vi "Tiempo.vi"() -> ()   [LabVIEW 2017]
panel:
  out "x-y":u32
  out "millisecond timer value 2":u32
  out "millisecond timer value":u32
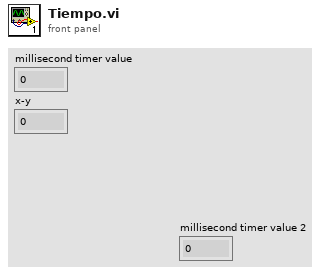
[diagram p1: front panel]
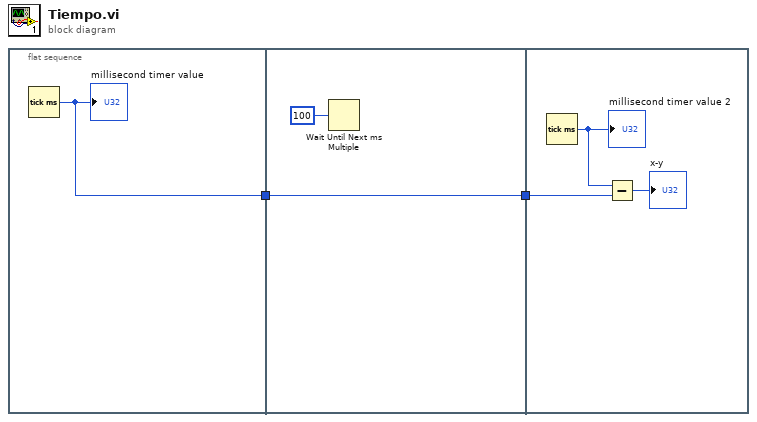
[diagram p0: block diagram]
diagram:
  n1 = flat-sequence {
    tunnel: [w3] -> w2
    tunnel: w2 -> [w5]
    tunnel: [w5] -> w1
    tunnel: w1 -> [w7]
    frame #0 {
      n2 = Tick Count (ms)() -> (millisecond timer value=w3:u32)
      "millisecond timer value" <- w3
    }
    frame #1 {
      n3 = Wait Until Next ms Multiple(millisecond multiple=u32 100) -> ()  [unwired: 1 out]
    }
    frame #2 {
      n4 = Tick Count (ms)() -> (millisecond timer value=w8:u32)
      "millisecond timer value 2" <- w8
      n5 = Subtract(x=w8, y=w7) -> (x-y=→"x-y":u32)
    }
  }
